vi "Velocidad por eje_V2.vi"(1 "Distancias centrales de las ruedas\n               configuración (m)":dbl[](array[numeric]), 3 "Frecuencia de muestreo":dbl, 4 "Puntos centrales de las ruedas\n             inductivo":sgl[](array[numeric])) -> (0 "Velocidad de eje":dbl[](array[numeric]))   [LabVIEW 2015]
doc: "Calcula la velocidad de cada eje"
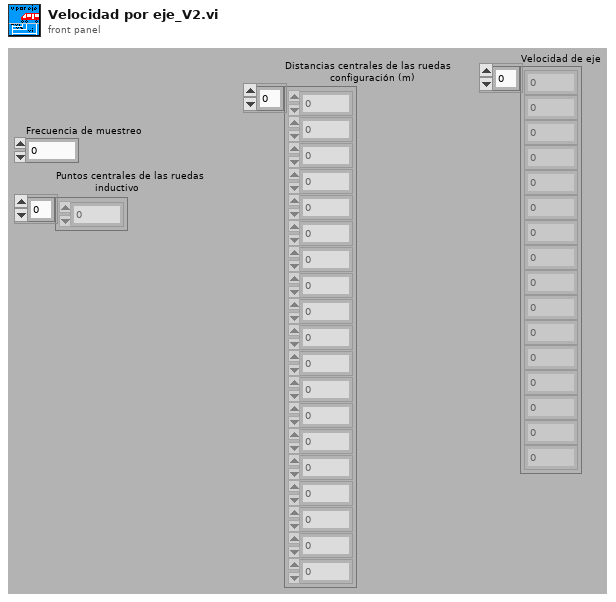
[diagram p1: front panel]
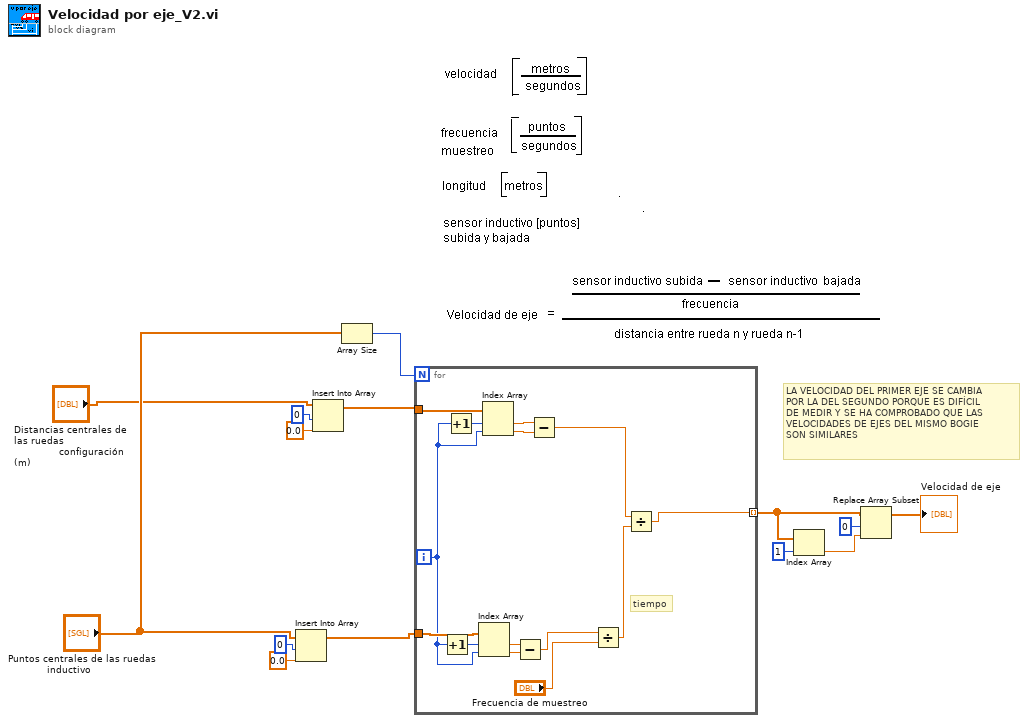
[diagram p0: block diagram]
diagram:
  # "LA VELOCIDAD DEL PRIMER EJE SE CAMBIA\nPOR LA DEL SEGUNDO PORQUE ES DIFÍCIL\nDE MEDIR Y SE HA COMPROBADO QUE LAS\nVELOCIDADES DE EJES DEL MISMO BOGIE \nSON SIMILARES"
  n1 = Insert Into Array(array="Puntos centrales de las ruedas\n             inductivo", index=0, new element=0.0 ("new element/subarray")) -> (w7:sgl[])
  n2 = Insert Into Array(array="Distancias centrales de las ruedas\n               configuración (m)", index=0, new element=0.0 ("new element/subarray")) -> (w11:dbl[])
  n3 = Array Size(array="Puntos centrales de las ruedas\n             inductivo") -> (size(s)=w14:i32)
  n4 = for {
    N: w14 -> [_]
    tunnel: w7 -> [w17]
    tunnel: w11 -> [w28]
    tunnel: [w21] -> w6 mode=indexing
    i -> [w15]
    # "tiempo"
    n5 = Increment(x=w15) -> (x+1=w20:i32)
    n6 = Increment(x=w15) -> (x+1=w27:i32)
    n7 = Index Array(array=w17, index #1=w20, index #2=w15) -> (element #1=w19:sgl, element #2=w18:sgl)
    n8 = Index Array(array=w28, index #1=w27, index #2=w15) -> (element #1=w25:dbl, element #2=w26:dbl)
    n9 = Subtract(x=w19, y=w18) -> (x-y=w16:sgl)
    n10 = Subtract(x=w25, y=w26) -> (x-y=w23:dbl)
    n11 = Divide(x=w16, y="Frecuencia de muestreo") -> (x/y=w22:dbl)
    n12 = Divide(x=w23, y=w22) -> (x/y=w21:dbl)
  }
  n13 = Index Array(array=w6, index=1) -> (element=w4:dbl)
  n14 = Replace Array Subset(array=w6, new element=w4, index=0) -> (→"Velocidad de eje":dbl[])
